vi "14to41.vi"(0 "QR50":i32[](array[numeric])) -> (1 "0":i32, 2 "1":i32, 3 "2":i32, 4 "3":i32)   [LabVIEW 2010]
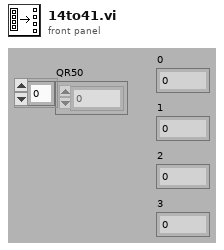
[diagram p1: front panel]
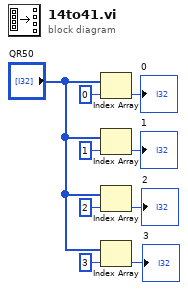
[diagram p0: block diagram]
diagram:
  n1 = Index Array(array="QR50", index=0) -> (element=→"0":i32)
  n2 = Index Array(array="QR50", index=1) -> (element=→"1":i32)
  n3 = Index Array(array="QR50", index=2) -> (element=→"2":i32)
  n4 = Index Array(array="QR50", index=3) -> (element=→"3":i32)
